vi "Calculate.vi"(7 "Conversion":refnum<k21>, 8 "error in (no error)":errorcluster, 9 "PCL dt":dbl, 10 "Values":dbl[](array[numeric]), 11 "Frame Configuration":T1 {"CRCConfiguration"."FinalXorValue" format="%0x"; "CRCConfiguration"."InitialCRC" format="%0x"; "CRCConfiguration"."Polynomial" format="%0x"; "CRC"."Data Type" items=["Signed", "Unsigned", "IEEE Float"]; "Rolling Counter"."Data Type" items=["Signed", "Unsigned", "IEEE Float"]; "Input Channels"."Data Type" items=["Signed", "Unsigned", "IEEE Float"]}) -> (0 "error out":errorcluster, 1 "ProtectionValue":dbl, 2 "Rolling Counter":dbl, 3 "Frame Configuration":T1 {"CRCConfiguration"."FinalXorValue" format="%0x"; "CRCConfiguration"."InitialCRC" format="%0x"; "CRCConfiguration"."Polynomial" format="%0x"; "CRC"."Data Type" items=["Signed", "Unsigned", "IEEE Float"]; "Rolling Counter"."Data Type" items=["Signed", "Unsigned", "IEEE Float"]; "Input Channels"."Data Type" items=["Signed", "Unsigned", "IEEE Float"]})   [LabVIEW 2021, in "LIN Frame Protection Addon Engine.lvlib"]
uses:
  LIN Frame Protection Addon Engine.lvlib
  Shared/Types/FrameConfiguration.ctl
  Shared/Types/InputChannelConfiguration.ctl
  Shared/Types/Protection Type.ctl
  Shared/Types/CRCConfiguration.ctl
  <vilib>/xnet/xnet.llb/XNET Convert (Signal to Frame Raw).vi
  Shared/LIN Frame Protection Addon Shared.lvlib
panel:
  out "PCLIterations":dbl
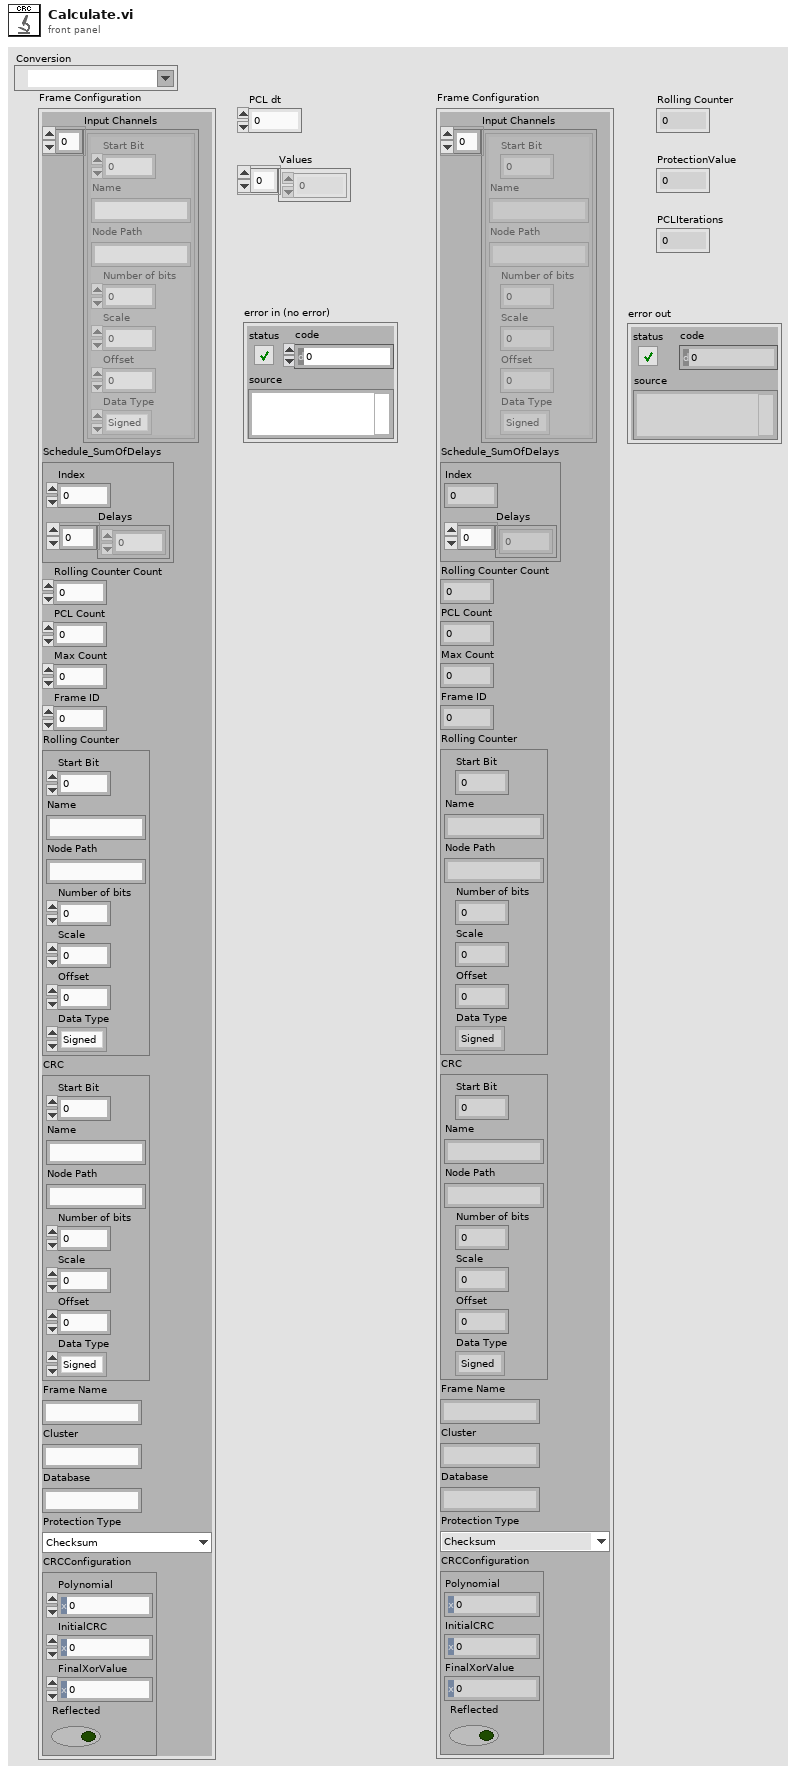
[diagram p1: front panel]
types:
  T1 = typedef "LIN Frame Protection Addon Shared.lvlib/FrameConfiguration.ctl" = cluster{"Input Channels":T2[], "Schedule_SumOfDelays":cluster{"Index":i32, "Delays":dbl[]}, "Rolling Counter Count":dbl, "PCL Count":u64, "Max Count":dbl, "Frame ID":u32, "Rolling Counter":T2, "CRC":T2, "Frame Name":string, "Cluster":string, "Database":string, "Protection Type":T3, "CRCConfiguration":T4}
  T2 = typedef "LIN Frame Protection Addon Shared.lvlib/InputChannelConfiguration.ctl" = cluster{"Start Bit":i32, "Name":string, "Node Path":string, "Number of bits":i32, "Scale":dbl, "Offset":dbl, "Data Type":u32}
  T3 = typedef "LIN Frame Protection Addon Shared.lvlib/Protection Type.ctl" = enum16{"Checksum", "CRC-8", "CRC-16", "CRC-32", "None (Counter Only)"}
  T4 = typedef "LIN Frame Protection Addon Shared.lvlib/CRCConfiguration.ctl" = cluster{"Polynomial":u64, "InitialCRC":u64, "FinalXorValue":u64, "Reflected":bool}
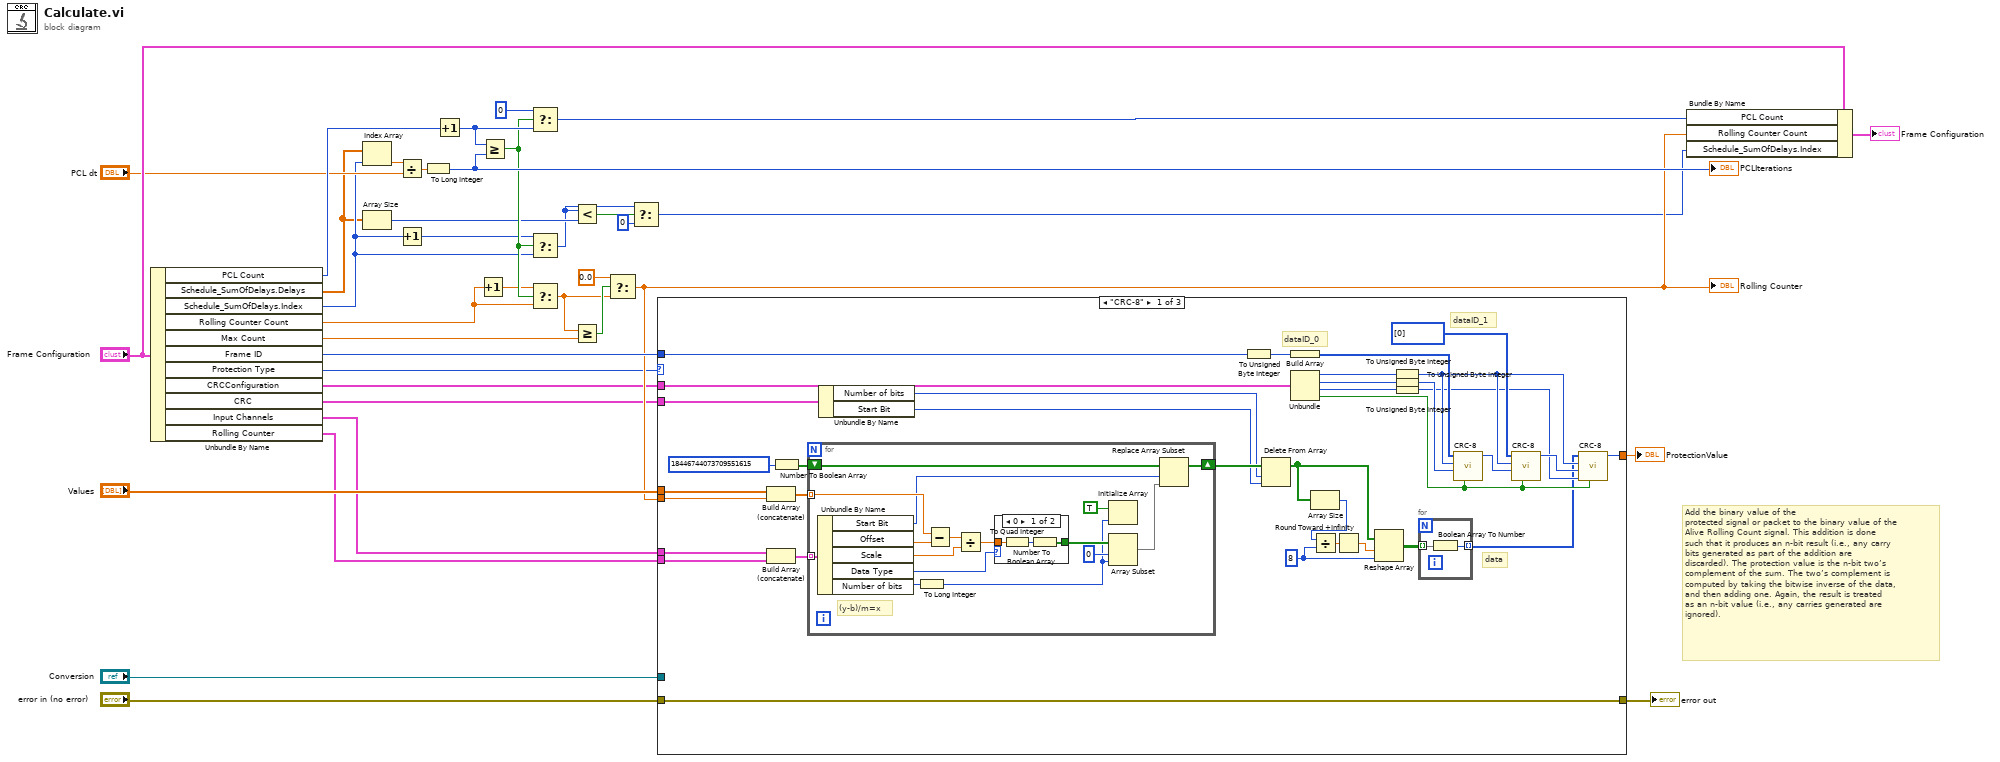
[diagram p0: block diagram]
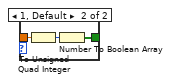
[diagram p2: hidden frame]
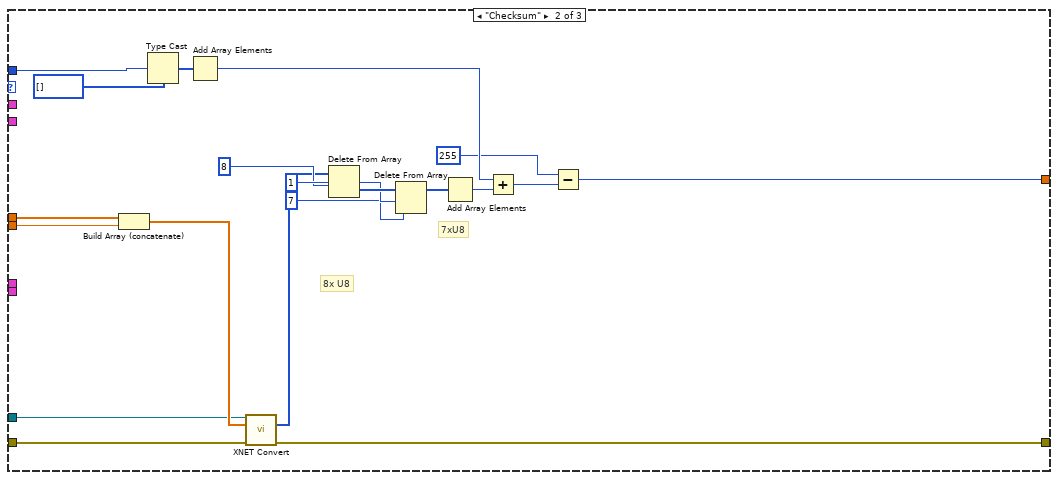
[diagram p3: hidden frame]
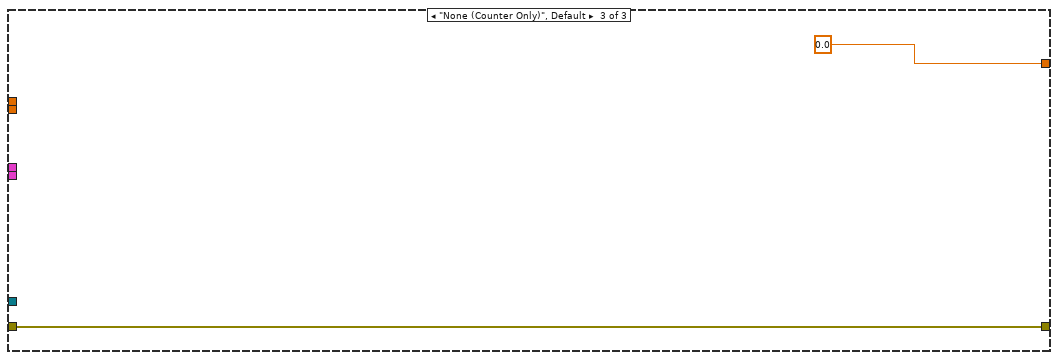
[diagram p4: hidden frame]
diagram:
  # "Add the binary value of the\nprotected signal or packet to the binary value of the\nAlive Rolling Count signal. This addition is done\nsuch that it produces an n-bit result (i.e., any carry\nbits generated as part of the addition are\ndiscarded). The protection value is the n-bit two’s\ncomplement of the sum. The two’s complement is\ncomputed by taking the bitwise inverse of the data,\nand then adding one. Again, the result is treated\nas an n-bit value (i.e., any carries generated are\nignored)."
  n1 = Unbundle By Name("Frame Configuration") -> ("PCL Count"=w34:u64, "Schedule_SumOfDelays.Delays"=w11:dbl[], "Schedule_SumOfDelays.Index"=w12:i32, "Rolling Counter Count"=w32:dbl, "Max Count"=w29:dbl, "Frame ID"=w24:u32, "Protection Type"=w17:T3, "CRCConfiguration"=w4:T4, "CRC"=w1:T2, "Input Channels"=w3:T2[], "Rolling Counter"=w2:T2)
  n2 = Index Array(array=w11, index=w12) -> (element=w16:dbl)
  n3 = Array Size(array=w11) -> (size(s)=w10:i32)
  n4 = Divide(x=w16, y="PCL dt") -> (x/y=w37:dbl)
  n5 = Increment(x=w12) -> (x+1=w8:i32)
  n6 = To Long Integer(number=w37) -> (32bit integer=w28:i32)
  "PCLIterations" <- w28
  n7 = Increment(x=w34) -> (x+1=w27:u64)
  n8 = Increment(x=w32) -> (x+1=w13:dbl)
  n9 = Greater Or Equal?(x=w27, y=w28) -> (x >= y?=w14:bool)
  n10 = Select(t=u64 0, s=w14, f=w27) -> (s? t:f=w25:u64)
  n11 = Select(t=w8, s=w14, f=w12) -> (s? t:f=w6:i32)
  n12 = Select(t=w13, s=w14, f=w32) -> (s? t:f=w15:dbl)
  n13 = Less?(x=w6, y=w10) -> (x < y?=w7:bool)
  n14 = Greater Or Equal?(x=w15, y=w29) -> (x >= y?=w36:bool)
  n15 = Select(t=0.0, s=w36, f=w15) -> (s? t:f=w21:dbl)
  "Rolling Counter" <- w21
  n16 = Select(t=w6, s=w7, f=0) -> (s? t:f=w5:i32)
  n17 = case shown="\"CRC-8\"" w17 {
    tunnel: w24 -> [w60 w110 _]
    tunnel: [w53 w105 0.0] -> w23
    tunnel: w3 -> [w72 _ _]
    tunnel: w2 -> [w71 _ _]
    tunnel: "Values" -> [w70 w104 _]
    tunnel: w21 -> [w69 w103 _]
    tunnel: "error in (no error)" -> [w64 w101 w118]
    tunnel: [w64 w100 w118] -> w19
    tunnel: "Conversion" -> [_ w99 _]
    tunnel: w4 -> [w63 _ _]
    tunnel: w1 -> [w43 _ _]
    frame "CRC-8" {
      w44 = 8 ("y")
      # "data"
      # "dataID_1"
      # "dataID_0"
      n18 = Build Array (concatenate)(w70, w69) -> (w68:dbl[])
      n19 = Build Array (concatenate)(w72, w71) -> (w65:T2[])
      n20 = Number To Boolean Array(number=u64 18446744073709551615) -> (Boolean array=w67:bool[])
      n21 = for {
        tunnel: w65 -> [w90] mode=indexing
        shift-right: [w81] -> w61
        shift-left: w67 -> [w83]
        tunnel: w68 -> [w80] mode=indexing
        # "(y-b)/m=x"
        n22 = Unbundle By Name(w90) -> ("Start Bit"=w77:i32, "Offset"=w89:dbl, "Scale"=w87:dbl, "Data Type"=w79:u32, "Number of bits"=w85:i32)
        n23 = To Long Integer(number=w85) -> (32bit integer=w76:i32)
        n24 = Subtract(x=w80, y=w89) -> (x-y=w88:dbl)
        n25 = Divide(x=w88, y=w87) -> (x/y=w86:dbl)
        n26 = case shown="0" w79 {
          tunnel: w86 -> [w93 w96]
          tunnel: [w91 w94] -> w78
          frame 0 {
            n27 = To Quad Integer(1:w93) -> (0:w92:i64)
            n28 = Number To Boolean Array(number=w92) -> (Boolean array=w91:bool[])
          }
          frame 1, Default {
            n29 = To Unsigned Quad Integer(1:w96) -> (0:w95:u64)
            n30 = Number To Boolean Array(number=w95) -> (Boolean array=w94:bool[])
          }
        }
        n31 = Initialize Array(TRUE ("Boolean"), w76) -> ()  [unwired: 1 out]
        n32 = Array Subset(array=w78, index=0, length=w76) -> (w82:bool[])
        n33 = Replace Array Subset(array=w83, new element=w82, index=w77) -> (w81:bool[])
      }
      n34 = Unbundle By Name(w43) -> ("Number of bits"=w38:i32, "Start Bit"=w39:i32)
      n35 = To Unsigned Byte Integer(number=w60) -> (unsigned 8bit integer=w59:u8)
      n36 = Delete From Array(array=w61, length=w38, index=w39) -> (array with subset deleted=w41:bool[])  [unwired: 1 out]
      n37 = Build Array(w59) -> (w58:u8[])
      n38 = Unbundle(w63) -> ("Polynomial"=w57:u64, "InitialCRC"=w62:u64, "FinalXorValue"=w54:u64, "Reflected"=w52:bool)
      n39 = Array Size(array=w41) -> (size(s)=w42:i32)
      n40 = Divide(x=w42, y=w44) -> (x/y=w47:dbl)
      n41 = Round Toward +Infinity(x=w47) -> (ceil(x): smallest int >= x=w45:dbl)
      n42 = Reshape Array(w41, w45, w44) -> (w46:bool[][])
      n43 = To Unsigned Byte Integer(number=w57) -> (unsigned 8bit integer=w50:u8)
      n44 = To Unsigned Byte Integer(number=w62) -> (unsigned 8bit integer=w49:u8)
      n45 = To Unsigned Byte Integer(number=w54) -> (unsigned 8bit integer=w48:u8)
      n46 = for {
        tunnel: w46 -> [w74] mode=indexing
        tunnel: [w73] -> w40 mode=indexing
        n47 = Boolean Array To Number(Boolean array=w74) -> (number=w73:u8)
      }
      n48 = call "CRC-8.vi"("Reflected"=w52, "InitialCRC"=w49, "Polynomial"=w50, "DATA"=w58) -> ("CRC"=w55:u8)  [unwired: 7 in]
      n49 = call "CRC-8.vi"("Reflected"=w52, "InitialCRC"=w55, "Polynomial"=w50, "DATA"=u8[] [0] ("Polynomial")) -> ("CRC"=w56:u8)  [unwired: 7 in]
      n50 = call "CRC-8.vi"("Reflected"=w52, "FinalXorValue"=w48, "InitialCRC"=w56, "Polynomial"=w50, "DATA"=w40) -> ("CRC"=w53:u8)  [unwired: 6 in]
    }
    frame "Checksum" {
      # "7xU8"
      # "8x U8"
      n51 = Build Array (concatenate)(w104, w103) -> (w102:dbl[])
      n52 = Type Cast(type=u8[] [], x=w110) -> (*(type *) &x=w109:u8[])
      n53 = Add Array Elements(numeric array=w109) -> (sum=w108:u8)
      n54 = call-poly <vilib>:"XNET Convert.vi"("session in"=w99, "signal data"=w102, "error in (no error)"=w101) -> ("frame data"=w97:u8[], "error out"=w100:errorcluster)  [unwired: 10 in, 1 out]
      n55 = Delete From Array(array=w97, length=8) -> (deleted portion=w116:u8[])  [unwired: 1 in, 1 out]
      n56 = Delete From Array(array=w116, length=1, index=7) -> (array with subset deleted=w113:u8[])  [unwired: 1 out]
      n57 = Add Array Elements(numeric array=w113) -> (sum=w112:u8)
      n58 = Add(x=w108, y=w112) -> (x+y=w107:u8)
      n59 = Subtract(x=u8 255, y=w107) -> (x-y=w105:u8)
    }
    frame "None (Counter Only)", Default {
    }
  }
  "ProtectionValue" <- w23
  "error out" <- w19
  n60 = Bundle By Name(cluster="Frame Configuration", "PCL Count"=w25, "Rolling Counter Count"=w21, "Schedule_SumOfDelays.Index"=w5) -> (→"Frame Configuration":T1)
